vi "Fake Create Client.vi"(8 "error in":errorcluster) -> (0 "error out":errorcluster, 3 "grpc client id":T1)   [LabVIEW 2020, in "MeasurementServerTests.lvlib" / "gRPC Utilities Tests.lvlib"]
uses:
  gRPC Utilities Tests.lvlib
  <vilib>/gRPC/LabVIEW gRPC Library/Shared/grpcId.ctl
  <vilib>/gRPC/LabVIEW gRPC Library/grpc-lvsupport-release.lvlib
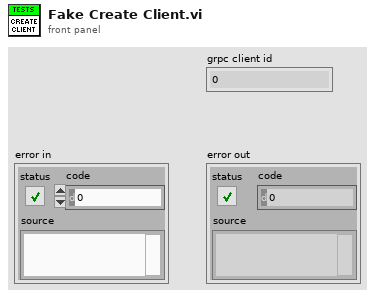
[diagram p1: front panel]
types:
  T1 = typedef "grpc-lvsupport-release.lvlib/grpcId.ctl" = u64
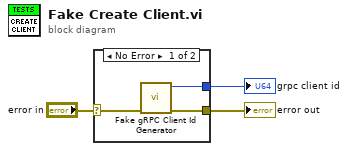
[diagram p0: block diagram]
diagram:
  n1 = case shown="No Error" "error in" {
    selector: "error in" -> [w6 w7]
    tunnel: [w5 w7] -> w2
    tunnel: [w4 _] -> w1
    frame No Error {
      n2 = call "Fake gRPC Client Id Generator.vi"("error in"=w6) -> ("error out"=w5:errorcluster, "client id"=w4:u64)  [unwired: 9 in]
    }
    frame Error {
    }
  }
  "grpc client id" <- w1
  "error out" <- w2
